vi "AlliGator Phasor Plot Mouse Move Event.vi"(7 "Source Image Display Refnum":T4, 8 "Error In":errorcluster, 9 "Current Phasor Plot Information Indicators":T6, 10 "Image User Event Data":T3, 11 "Alligator Queue Elements in":T1[](array[typedef])) -> (0 "Error Out":errorcluster, 3 "AlliGator Queue Elements out":T1[](array[typedef]))   [LabVIEW 2021, in "AlliGator Phasor Plot.lvlib"]
doc: "Handles mouse move events in the Phasor Plot image."
uses:
  AlliGator Phasor Plot.lvlib
  GUI/AlliGator Phasor Plot Ctrl Refnums.ctl
  Image/Image Control Refnum.ctl
  Image/Image Display User Event Data.ctl
  <vilib>/Utility/miscctls.llb/LVPoint32TypeDef.ctl
  Action Engine/AlliGator Q Element.ctl
  Action Engine/AlliGator Q Event.ctl
  Action Engine/Alligator Elements Order in Action Stack.ctl
  Utilities/Read-Write.ctl
  Phasor Ratio/AlliGator Phasor Reference Data.ctl
  034bdac3-b367-4aff-a885-c1a04e73f031.vi
  034bdac3-b367-4aff-a885-c1a04e73f031.vi/539bd7ec-d9e8-460f-a56d-a449b4a86a5e.vi
  Action Engine/AlliGator Add Action Array to Stack.vi
  Action Engine/AlliGator Action Engine.lvlib
  Phasor Ratio/AlliGator Phasor Ratio.lvlib
  GUI/GUI.lvlib
  Utilities/Utilities.lvlib
  GUI/AlliGator GUI.lvlib
  Image/Image.lvlib
panel:
  # "see the AlliGator License on the block diagram (Ctrl+E or Window:Show Block Diagram)"
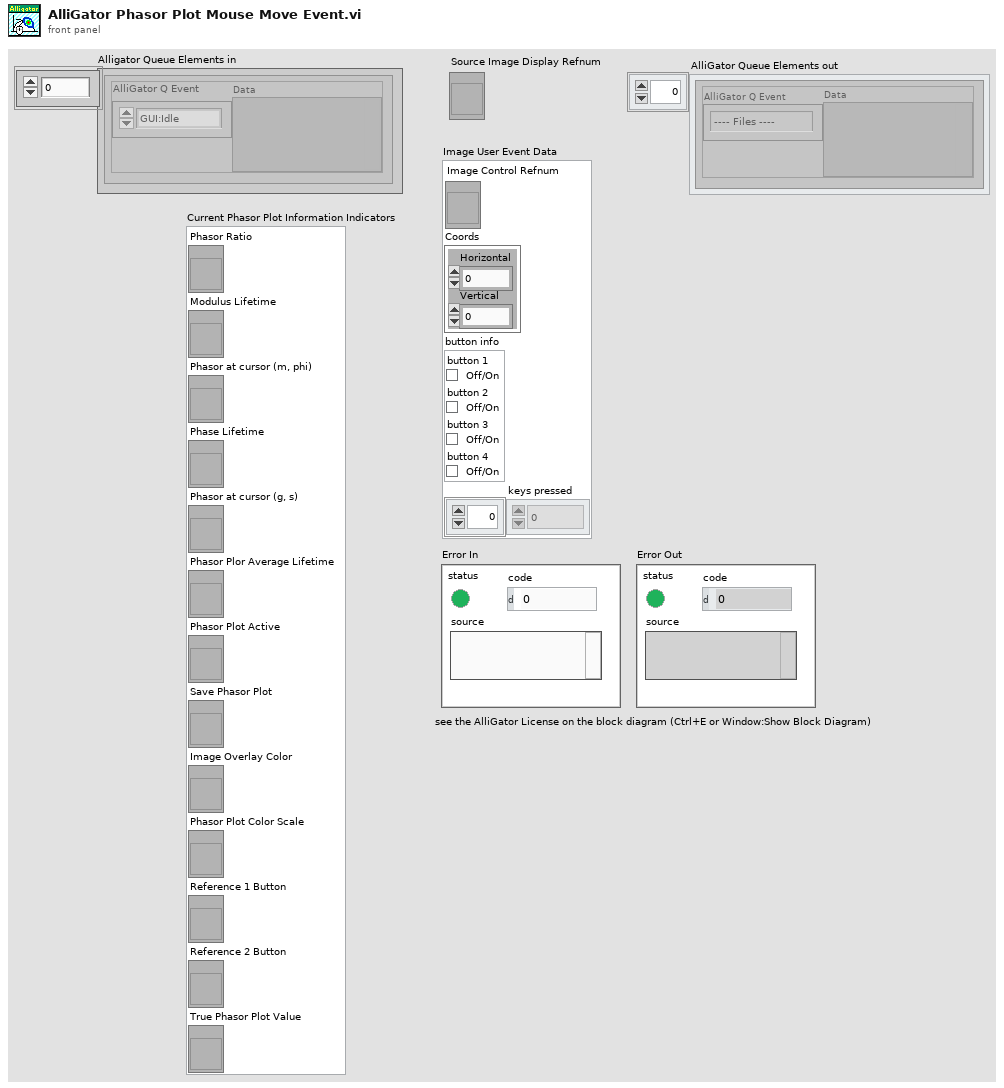
[diagram p1: front panel]
types:
  T1 = typedef "AlliGator Action Engine.lvlib/AlliGator Q Element.ctl" = cluster{"AlliGator Q Event":T2, "Data":variant}
  T2 = typedef "AlliGator Action Engine.lvlib/AlliGator Q Event.ctl" = enum16{"---- Files ----", "Files:Set Batch Export Files To Save", "Files:Set Dataset Loading & Pre-processing Options", "Files:Check #Frames in Dataset", "Files:Increment Frame Index", "Files:Open Mask Image", "Files:Open White Light Image", "Files:Open Single Dataset", "Files:New Folder of Folders Selected", "Files:Load File (all Types)_Scriptable", "Files:Move Flattened Series to Folders Series", "Files:Select Folder", "Files:Load FLI Dataset", "Files:Load Swiss SPAD 1 Dataset", "Files:Load Swiss SPAD 2 Dataset", "Files:Load .sdt FLI Dataset", "Files:Load .ptu FLI Dataset", "Files:Load .bin FLI Dataset", "Files:Load Single Gate Image Folder", "Files:Load I/m/phi Dataset (deprecated)", "Files:Load Single Image", "Files:Subtract Background File", "Files:Export FLI Dataset", "Files:Load HDF5 FLI Dataset", "Files:Set Destination File Path", "Files:Save Mask Image", "Files:Batch Conversion", "Files:New Folder Selected", "Files:Close FLI Dataset", "Files:Close FLI Dataset Series", "Files:Close White Light Image", "Files:Close Mask Image", "---- FLI Dataset ----", "FLI Dataset:Channel Arithmetic", "FLI Dataset:Export Average Lifetime Map as ASCII", "FLI Dataset:Export User-Defined Quantity Map as ASCII", "FLI Dataset:Python Function FLI Dataset Event", "FLI Dataset:ROI Analysis", "FLI Dataset:Tilted Logistic Square Gated IRF Characteristics Map", "FLI Dataset:Logistic Square Gated IRF Characteristics Map", "FLI Dataset:Square Gated IRF Characteristics Map", "FLI Dataset:Multi-ROI Single-Pixel Phasor Analysis", "FLI Dataset:Multi-ROI Single-Pixel NLSF Analysis", "FLI Dataset:All ROIs IRF Extraction", "FLI Dataset:All ROIs Decay Fit Non-Interactive (Fast + Individual IRF)", "FLI Dataset:All ROIs Phasor Analysis", "FLI Dataset:All ROIs Decay Fit", "FLI Dataset:Fluorescence Decay Statistics", "FLI Dataset:Update Decay Statistics Graph", "FLI Dataset:Get Decay from ROI", "FLI Dataset:All ROIs Average Lifetimes", "FLI Dataset:Save/Load Local IRFs", "FLI Dataset:Clear Local IRFs", "FLI Dataset:Phasor Calibration Maps (# Gates Series) Script", "FLI Dataset:Calibrated Phasor Map Series", "---- FLI Dataset Series ----", "FLI Dataset Series:Sum All Datasets in Series", "FLI Dataset Series:Add Dataset to Accumulated Dataset", "FLI Dataset Series:Display Accumulated Dataset", "FLI Dataset Series:Clear Dataset Series Sum", "FLI Dataset Series:Time-Series Analysis (NLSF)", "FLI Dataset Series:Time-Series Analysis (Phasor)", "---- Image ----", "Image:Update Image Profile Plots", "Image:Image Histogram Cursor Move", "Image:Image Histogram", "Image:Image Contrast", "Image:Set Image Histogram Cursor Move Flag", "Image:Clear Image Overlay", "Image:Use ROI as Search Area", "Image:Set ROI Diameter", "Image:Save Image Data as TIFF", "Image:Save Displayed Image with Overlay", "Image:Save Image Overlay Only", "Image:Save Image as Hot Pixel Mask", "Image:Change Source Image Color Palette", "Image:Copy Image to Clipboard", "Image:Source Image ROI Selection", "Image:Delete All ROIs", "Image:Delete All Unselected ROIs", "Image:Delete ROI", "Image:Merge All ROIs", "Image:Store ROI", "Image:Source Image ROI Storage", "Image:Export ROI Description to Notebook", "Image:Save ROI", "Image:Load ROI", "Image:Paste ROI Definition", "Image:Clear ROI", "Image:Identify ROIs in Mask Image", "Image:Create Complementary ROI", "Image:Create Contour ROI", "Image:Create ROI(s) from Pixels with Peak above Min_Scriptable", "Image:Create ROI(s) from Pixels with Intensity above Min_Scriptable", "Image:Compute ROI Statistics", "Image:Delete ROI(s) based on ROI Characteristics", "Image:Create ROI Grid", "Image:ROI to Individual Pixel ROIs", "Image:Python Function Source Image Event", "Image:Show Phasor Calibration Map ROI Centers", "Image:Convert ROI to Mask Image", "Image:Mouse Move", "Image:Mouse Up", "Image:Set Source Image Mouse Move Flag", "Image:Add Scale Bar Overlay", "Image:Delete Existing ROIs Option", "Image:Overlay ROI Median", "Image:Check Current ROI", "Image:Update True Pixel Value", "---- Decay ----", "Decay:Clear IRF/Reference Plot", "Decay:Add Decay to Graph", "Decay:Smoothen Plot", "Decay:Smoothen Plot Tail", "Decay:Average Selected Plots", "Decay:Extract IRF", "Decay:Optimal IRF Extraction", "Decay:Threshold IRF", "Decay:Fit to Model IRF", "Decay:Fit IRF to Square Gate", "Decay:Fit IRF to Logistic Square Gate", "Decay:Fit IRF to Tilted Logistic Square Gate", "Decay:Create Bounding Cursors Set", "Decay:Export Bounding Cursors Definition to Notebook", "Decay:Denoise Plot", "Decay:Compute Cumulative Function", "Decay:Use as Reference Decay", "Decay:Show Reference Decay/IRF", "Decay:Extrapolate Decay", "Decay:Create Head & Tail Bounding Cursors", "Decay:Store Cursor-defined Head & Tail Fractions", "Decay:Rebin Plot", "Decay:1-Normalize Decay", "Decay:[0-1]-Normalize Plot", "Decay:Straighten Decay", "Decay:Shift Decay", "Decay:Fold Decay", "Decay:Fit Decay", "Decay:Global Fit of Selected Decays", "Decay:Post Global Fit Script", "Decay:Add Global Fit Parameters to Graph", "Decay:Add Decay Parameter(s) to Plot (Graph)", "Decay:Export Decay to Phasor Graph", "Decay:Compute Average Lifetime", "Decay:Plot Convolution", "Decay:Graph Tip Strip Update", "---- Decay Statistics ----", "Decay Statistics:Tip Strip Update", "---- Intensity Time Trace ----", "Intensity Time Trace:Use File Timestamp", "Intensity Time Trace:Load Intensity Corrections File", "Intensity Time Trace:Clear Intensity Corrections File", "Intensity Time Trace:Tip Strip Update", "---- Phasor Plot ----", "Phasor Plot:Build Phasor Plot", "Phasor Plot:Change Phasor Plot Color Palette", "Phasor Plot:Adjust Phasor Plot Display Range", "Phasor Plot:Highlight Image ROI in Phasor Plot", "Phasor Plot:Save Phasor Plot Image with Overlay", "Phasor Plot:Export Complex Phasor Map", "Phasor Plot:Export Phasor Ratio Map", "Phasor Plot:Export Average Lifetime Map", "Phasor Plot:Compute Phase Lifetime Histogram", "Phasor Plot:Compute Phasor Ratio Histogram", "Phasor Plot:Compute Phase Lifetime vs Intensity Scatter Plot", "Phasor Plot:Weber 2-Component Decomposition", "Phasor Plot:Update Phasor Color Map Vertices", "Phasor Plot:Clear Phasor Overlay", "Phasor Plot:Use Segment Extremities as References", "Phasor Plot:Use UC/Segment Intersections as References", "Phasor Plot:Use UC/Principal Axis Intersections as References", "Phasor Plot:Use UC/Linear Fit Intersections as References", "Phasor Plot:Update Phasor Plot Reference", "Phasor Plot:Show Local Phasor Info in Phasor Plot", "Phasor Plot:Update Phasor Plot State", "Phasor Plot:Phasor Plot ROI Storage", "Phasor Plot:Phasor Plot ROI Selection", "Phasor Plot:Python Function Phasor Plot Event", "Phasor Plot:Overlay Phasor ROI, Ratio or Map in Source Image", "Phasor Plot:Compute Decay of Selected Phasors", "Phasor Plot:Phasor at Image Pixel", "Phasor Plot:Mouse Move", "Phasor Plot:Mouse Up", "Phasor Plot:Display Range Mouse Move", "Phasor Plot:Set Mouse Move Flag", "Phasor Plot:Update True Phasor Plot Value", "---- Phasor Graph ----", "Phasor Graph:Get Phasor Value", "Phasor Graph:Create New Phasor Plot Dialog", "Phasor Graph:Update Last Phasor Value", "Phasor Graph:Update Phasor (m, phi)", "Phasor Graph:Remove Single Phasor from Plot", "Phasor Graph:Add Single Phasor to Plot", "Phasor Graph:Remove Phasor Plot", "Phasor Graph:Remove Selected Phasor Plots", "Phasor Graph:Clear Phasor Data", "Phasor Graph:Clear Phasor Graph", "Phasor Graph:Cursor Move", "Phasor Graph:Draw Cursor Connecting Line", "Phasor Graph:Clear Cursor Connecting Line", "Phasor Graph:Find UC Intersection", "Phasor Graph:Use UC/Cursor-Defined Line Intersections", "Phasor Graph:Use Selected Plots Fitted Line/UC Intersections", "Phasor Graph:Use Selected Plots Principal Axis/UC Intersections", "Phasor Graph:Show Single Phasor", "Phasor Graph:Save Single Phasor Plot", "Phasor Graph:Save All Phasor Plots", "Phasor Graph:Load Phasor Plot(s)", "Phasor Graph:Phasor Multiplication", "Phasor Graph:Compute Average Phasor", "Phasor Graph:Compute Multiple Average Phasors (Selected Plots)", "Phasor Graph:Export Single Phasor Plot Phase Lifetimes", "Phasor Graph:Parameter 2 vs Parameter 1 Scatter Plot", "Phasor Graph:Use Cursor n Location", "Phasor Graph:Set Reference n to Current Phase Lifetime Value", "Phasor Graph:Set Reference n to Lifetime Value", "Phasor Graph:Set Cursor n Location", "Phasor Graph:Save Phasor Graph Image", "Phasor Graph:Update SEPL Plot", "Phasor Graph:Export Single Phasor Plot Data", "Phasor Graph:Export Selected Phasor Plots Data", "Phasor Graph:Python Function Phasor Graph Event", "Phasor Graph:Tip Strip Update", "---- Calibration ----", "Calibration:Set Calibration Type", "Calibration:Load/Save Phasor Calibration", "Calibration:Load/Save Phasor Calibration Series", "Calibration:Load/Save Phasor Calibration Map", "Calibration:Use as Calibration", "Calibration:Compute Optimal Calibration from Phasor References", "Calibration:Clear Phasor Calibration", "Calibration:Single Phasor Calibration Information", "Calibration:Use as Calibration Series", "Calibration:Use as Calibration Map", "Calibration:Clear Calibration Series", "Calibration:Phasor Calibration Series Information", "Calibration:Clear Calibration Map", "Calibration:Phasor Calibration Map Information", "Calibration:Apply Phasor Calibration", "Calibration:Update Single Plot Calibration", "Calibration:Update Multiple Plots Calibration", "Calibration:Clear Single Plot Calibration", "Calibration:Clear All Plots Calibrations", "Calibration:Clear Plot(s) Calibration(s)?", "---- Phasor Ratio ----", "Phasor Ratio:Clear Reference n", "Phasor Ratio:Toggle Selected Plot(s)  Lock to Reference 1", "Phasor Ratio:Use as Reference n", "Phasor Ratio:Send Reference n to Notebook", "Phasor Ratio:Toggle Selected Plot(s)  Lock to Reference 2", "Phasor Ratio:Compute Phasor Ratio at Mouse Location", "Phasor Ratio:Compute Phasor Plot's Average Phasor Ratio", "Phasor Ratio:Compute Time-Series Phasor Ratios", "Phasor Ratio:Fit Line to Phasor Ratio Plot", "Phasor Ratio:Save References", "Phasor Ratio:Load References", "Phasor Ratio:Update Phasor Reference 1", "Phasor Ratio:Update Phasor Reference 2", "Phasor Ratio:Move Cursor n to Reference n", "Phasor Ratio:Use as Phasor Reference 1 Lifetime", "Phasor Ratio:Use as Phasor Reference 2 Lifetime", "Phasor Ratio:Export Phasor Ratio Map as ASCII", "Phasor Ratio:Tip Strip Update", "---- Lifetime & Other Parameters Graph ----", "Lifetime:Compute Sliced Mean, SDV and CV Plots", "Lifetime:Plot Decay Shifts", "Lifetime:Plot Histogram", "---- Decay Fit Parameter Map ----", "Decay Fit Parameter Map:Export ROI NLSF Data as ASCII", "Decay Fit Parameter Map:Set Decay Fit Parameter Map Selection", "Decay Fit Parameter Map:Build Decay Fit Parameter Map", "Decay Fit Parameter Map:Change Decay Fit Parameter Map Color Palette", "Decay Fit Parameter Map:Export Decay Fit Parameter Map Data as ASCII", "Decay Fit Parameter Map:Export All Decay Fit Parameter Maps Data as ASCII", "Decay Fit Parameter Map:Selected Parameter Scatterplot", "Decay Fit Parameter Map:Parameter 2 vs Parameter 1 Scatterplot", "Decay Fit Parameter Map:Save Decay Fit Parameter Map Image", "Decay Fit Parameter Map:Save-Load IRFs & Fit Data", "Decay Fit Parameter Map:Update Local Decay Plots", "Decay Fit Parameter Map:Python Function Decay Fit Parameters Map Event", "Decay Fit Parameter Map:Overlay Decay Fit Parameter Map in Source Image", "Decay Fit Parameter Map:Selected Parameter vs Intensity Scatterplot", "Decay Fit Parameter Map:Mouse Up", "Decay Fit Parameter Map:Mouse Move", "Decay Fit Parameter Map:Display Range Mouse Move", "Decay Fit Parameter Map:Change Map Resolution", "Decay Fit Parameter Map:Variance Significance Maps", "Decay Fit Parameter Map:Fit Result Constraints Window", "---- Parameter Map ----", "Parameter Map:Export ROI Parameters Data as ASCII", "Parameter Map:Add Parameter Map Set", "Parameter Map:Delete Parameter Map Set", "Parameter Map:Update Parameter List", "Parameter Map:Build Parameter Map", "Parameter Map:Change Parameter Map Color Palette", "Parameter Map:Export Parameter Map Data as ASCII", "Parameter Map:Export All Parameter Maps Data as ASCII", "Parameter Map:Selected Parameter Scatterplot", "Parameter Map:Parameter 2 vs Parameter 1 Scatterplot", "Parameter Map:Selected Parameter vs Intensity Scatterplot", "Parameter Map:Save Parameter Map Image", "Parameter Map:Save-Load IRFs & Parameter Maps (TODO)", "Parameter Map:Set Parameter Map Selection", "Parameter Map:Python Function Parameter Map Event", "Parameter Map:Overlay Parameter Map in Source Image", "Parameter Map:Update Local Decay Plots", "Parameter Map:Mouse Up", "Parameter Map:Mouse Move", "Parameter Map:Display Range Mouse Move", "---- Generic Graph ----", "Generic Graph:Generic XY Graph Event", "Generic Graph:Python Function XY Graph Event", "Generic Graph:New Plot", "Generic Graph:Save Plot", "Generic Graph:XY Plot Histogram", "Generic Graph:Set XY Graph Plot Name", "Generic Graph:Set Last Cursor Style", "Generic Graph:Tip Strip Update", "---- GUI ----", "GUI:Start Script", "GUI:Type of Displayed Image Changed", "GUI:Gate Image Slide Changed", "GUI:Show Busy Icon", "GUI:Show Busy Icon & Abort Button", "GUI:Hide Busy Icon", "GUI:Hide Busy Icon & Abort Button", "GUI:Abort", "GUI:End Script", "GUI:Start Timing", "GUI:End Timing", "GUI:Set State Indicator", "GUI:Send Parameters JSON Strings to Clipboard", "GUI:Set Gate Step", "GUI:Idle", "GUI:Initialization", "GUI:Quit", "GUI:Increment Dataset Index", "GUI:Set Dataset Index to -1", "GUI:Time Series Slider Moved", "GUI:Time Series Slider Changed", "GUI:Toggle Playback or Loop", "GUI:Playback Script", "GUI:Set Phasor Frequency", "GUI:Open Window", "GUI:Start Test Script", "GUI:End Test Script", "GUI:Set Verbose Mode", "GUI:Set Verbose Settings Mode", "DEBUG"}
  T3 = typedef "Image.lvlib/Image Display User Event Data.ctl" = cluster{"Image Control Refnum":T4, "Coords":T5, "button info":cluster{"button 1":bool, "button 2":bool, "button 3":bool, "button 4":bool}, "keys pressed":enum16{"0", "1", "2", "3", "4", "5", "6", "7", "8", "9", "A", "B", "C", "D", "E", "F", "G", "H", "I", "J", "K", "L", "M", "N", "O", "P", "Q", "R", "S", "T", "U", "V", "W", "X", "Y", "Z", "F1", "F2", "F3", "F4", "F5", "F6", "F7", "F8", "F9", "F10", "F11", "F12", "F13", "F14", "F15", "ADD", "BACK", "BACKSLASH", "CAPITAL", "COMMA", "DECIMAL", "DELETE", "DIVIDE", "DOWN", "END", "EQUALS", "ESCAPE", "GRAVE (`)", "HOME", "INSERT", "LBRACKET", "LCONTROL", "LEFT", "L ALT", "LSHIFT", "LWIN", "MINUS", "MULTIPLY", "NEXT", "NUMLOCK", "NUMPAD_0", "NUMPAD_1", "NUMPAD_2", "NUMPAD_3", "NUMPAD_4", "NUMPAD_5", "NUMPAD_6", "NUMPAD_7", "NUMPAD_8", "NUMPAD_9", "PAUSE", "PERIOD", "PRIOR (PG UP)", "RBRACKET", "RCONTROL", "RETURN", "RIGHT", "R ALT", "RSHIFT", "RWIN", "SCROLL", "SEMICOLON", "SLASH", "SPACE", "SUBTRACT", "TAB", "UP", "ENTER (num pad)", "' (quote)"}[]}
  T4 = typedef "Image.lvlib/Image Control Refnum.ctl" = refnum<vi>
  T5 = typedef "LVPoint32TypeDef.ctl" = cluster{"Horizontal":i32, "Vertical":i32}
  T6 = typedef "AlliGator GUI.lvlib/AlliGator Phasor Plot Ctrl Refnums.ctl" = cluster{"Phasor Ratio":refnum<vi>, "Modulus Lifetime":refnum<vi>, "Phasor at cursor (m, phi)":refnum<vi>, "Phase Lifetime":refnum<vi>, "Phasor at cursor (g, s)":refnum<vi>, "Phasor Plor Average Lifetime":refnum<vi>, "Phasor Plot Active":refnum<vi>, "Save Phasor Plot":refnum<vi>, "Image Overlay Color":refnum<vi>, "Phasor Plot Color Scale":refnum<vi>, "Reference 1 Button":refnum<vi>, "Reference 2 Button":refnum<vi>, "True Phasor Plot Value":refnum<vi>}
  T7 = typedef "AlliGator Action Engine.lvlib/Alligator Elements Order in Action Stack.ctl" = enum16{"Enqueue 2 AFTER 1", "Enqueue 2 BEFORE 1"}
  T8 = enum16{"0", "1", "2", "3", "4", "5", "6", "7", "8", "9", "A", "B", "C", "D", "E", "F", "G", "H", "I", "J", "K", "L", "M", "N", "O", "P", "Q", "R", "S", "T", "U", "V", "W", "X", "Y", "Z", "F1", "F2", "F3", "F4", "F5", "F6", "F7", "F8", "F9", "F10", "F11", "F12", "F13", "F14", "F15", "ADD", "BACK", "BACKSLASH", "CAPITAL", "COMMA", "DECIMAL", "DELETE", "DIVIDE", "DOWN", "END", "EQUALS", "ESCAPE", "GRAVE (`)", "HOME", "INSERT", "LBRACKET", "LCONTROL", "LEFT", "L ALT", "LSHIFT", "LWIN", "MINUS", "MULTIPLY", "NEXT", "NUMLOCK", "NUMPAD_0", "NUMPAD_1", "NUMPAD_2", "NUMPAD_3", "NUMPAD_4", "NUMPAD_5", "NUMPAD_6", "NUMPAD_7", "NUMPAD_8", "NUMPAD_9", "PAUSE", "PERIOD", "PRIOR (PG UP)", "RBRACKET", "RCONTROL", "RETURN", "RIGHT", "R ALT", "RSHIFT", "RWIN", "SCROLL", "SEMICOLON", "SLASH", "SPACE", "SUBTRACT", "TAB", "UP", "ENTER (num pad)", "' (quote)"}[]
  T9 = enum16{"0", "1", "2", "3", "4", "5", "6", "7", "8", "9", "A", "B", "C", "D", "E", "F", "G", "H", "I", "J", "K", "L", "M", "N", "O", "P", "Q", "R", "S", "T", "U", "V", "W", "X", "Y", "Z", "F1", "F2", "F3", "F4", "F5", "F6", "F7", "F8", "F9", "F10", "F11", "F12", "F13", "F14", "F15", "ADD", "BACK", "BACKSLASH", "CAPITAL", "COMMA", "DECIMAL", "DELETE", "DIVIDE", "DOWN", "END", "EQUALS", "ESCAPE", "GRAVE (`)", "HOME", "INSERT", "LBRACKET", "LCONTROL", "LEFT", "L ALT", "LSHIFT", "LWIN", "MINUS", "MULTIPLY", "NEXT", "NUMLOCK", "NUMPAD_0", "NUMPAD_1", "NUMPAD_2", "NUMPAD_3", "NUMPAD_4", "NUMPAD_5", "NUMPAD_6", "NUMPAD_7", "NUMPAD_8", "NUMPAD_9", "PAUSE", "PERIOD", "PRIOR (PG UP)", "RBRACKET", "RCONTROL", "RETURN", "RIGHT", "R ALT", "RSHIFT", "RWIN", "SCROLL", "SEMICOLON", "SLASH", "SPACE", "SUBTRACT", "TAB", "UP", "ENTER (num pad)", "' (quote)"}
  T10 = typedef "Utilities.lvlib/Read-Write.ctl" = enum16{"Read", "Write"}
  T11 = typedef "AlliGator Phasor Ratio.lvlib/AlliGator Phasor Reference Data.ctl" = cluster{"Data Type":string, "Data":variant}
  T12 = typedef "IMAQ Image.ctl" = refnum<image>
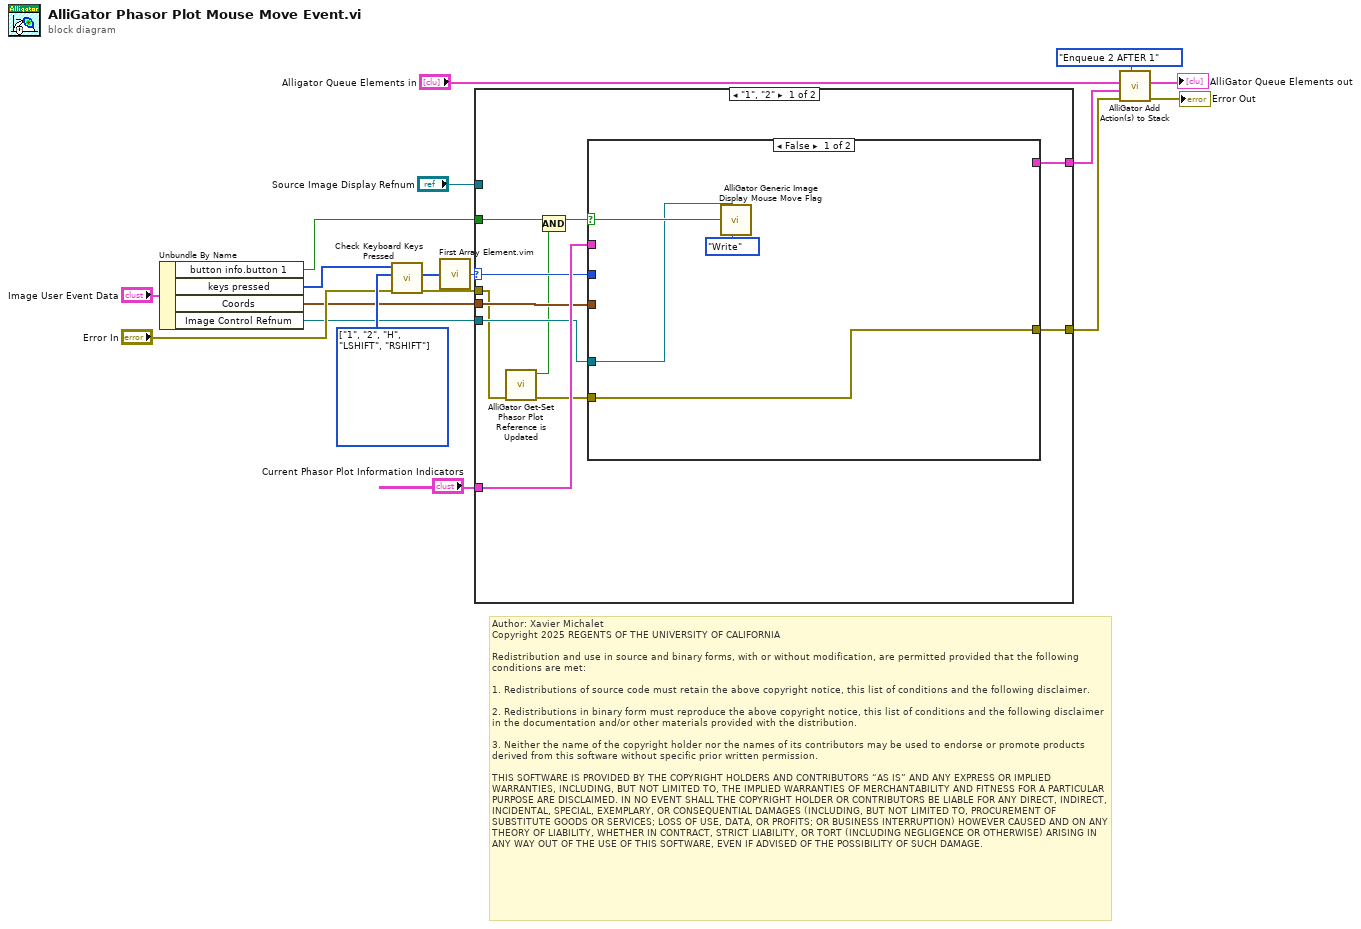
[diagram p0: block diagram]
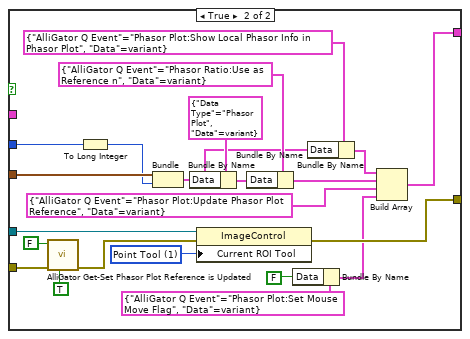
[diagram p2: hidden frame]
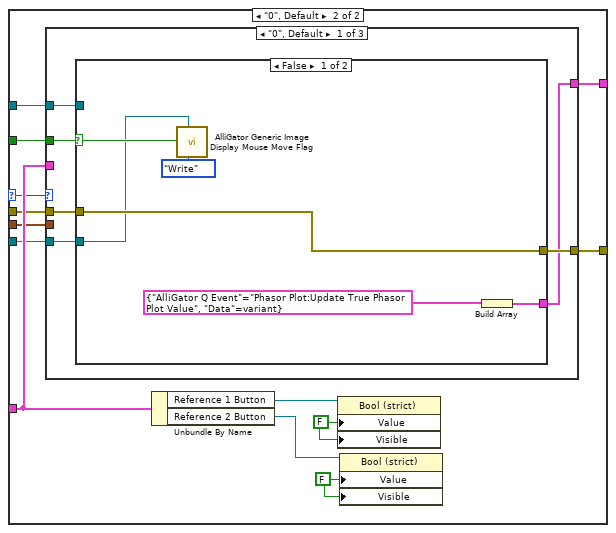
[diagram p3: hidden frame]
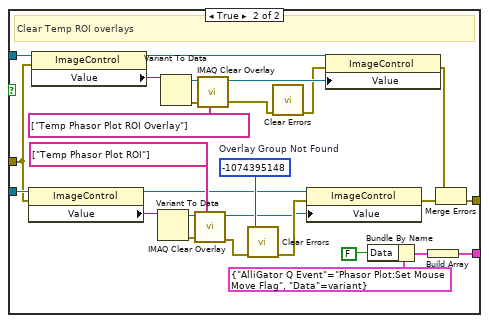
[diagram p4: hidden frame]
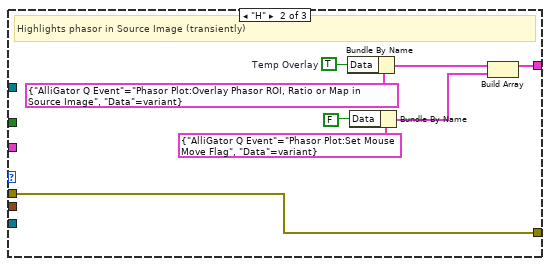
[diagram p5: hidden frame]
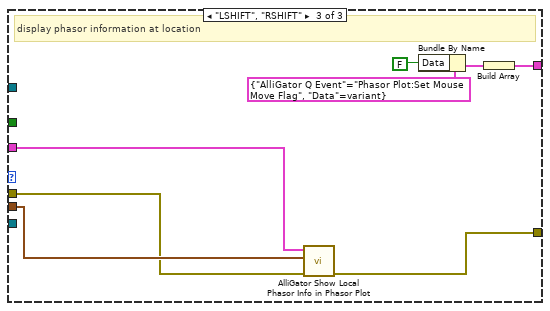
[diagram p6: hidden frame]
diagram:
  w17 = T8 [enum."1", enum."2", enum."H", enum."LSHIFT", enum."RSHIFT"] items=["0", "1", "2", "3", "4", "5", "6", "7", "8", "9", "A", "B", "C", "D", "E", "F", "G", "H", "I", "J", "K", "L", "M", "N", "O", "P", "Q", "R", "S", "T", "U", "V", "W", "X", "Y", "Z", "F1", "F2", "F3", "F4", "F5", "F6", "F7", "F8", "F9", "F10", "F11", "F12", "F13", "F14", "F15", "ADD", "BACK", "BACKSLASH", "CAPITAL", "COMMA", "DECIMAL", "DELETE", "DIVIDE", "DOWN", "END", "EQUALS", "ESCAPE", "GRAVE (`)", "HOME", "INSERT", "LBRACKET", "LCONTROL", "LEFT", "L ALT", "LSHIFT", "LWIN", "MINUS", "MULTIPLY", "NEXT", "NUMLOCK", "NUMPAD_0", "NUMPAD_1", "NUMPAD_2", "NUMPAD_3", "NUMPAD_4", "NUMPAD_5", "NUMPAD_6", "NUMPAD_7", "NUMPAD_8", "NUMPAD_9", "PAUSE", "PERIOD", "PRIOR (PG UP)", "RBRACKET", "RCONTROL", "RETURN", "RIGHT", "R ALT", "RSHIFT", "RWIN", "SCROLL", "SEMICOLON", "SLASH", "SPACE", "SUBTRACT", "TAB", "UP", "ENTER (num pad)", "' (quote)"] ("key targets (all)")
  # "Author: Xavier Michalet\nCopyright 2025 REGENTS OF THE UNIVERSITY OF CALIFORNIA\n\nRedistribution and use in source and binary forms, with or without modification, are permitted provided that the following conditions are met:\n\n1. Redistributions of source code must retain the above copyright notice, this list of conditions and the following disclaimer.\n\n2. Redistributions in binary form must reproduce the above copyright notice, this list of conditions and the following disclaimer in the documentation and/or other materials provided with the distribution.\n\n3. Neither the name of the copyright holder nor the names of its contributors may be used to endorse or promote products derived from this software without specific prior written permission.\n\nTHIS SOFTWARE IS PROVIDED BY THE COPYRIGHT HOLDERS AND CONTRIBUTORS “AS IS” AND ANY EXPRESS OR IMPLIED WARRANTIES, INCLUDING, BUT NOT LIMITED TO, THE IMPLIED WARRANTIES OF MERCHANTABILITY AND FITNESS FOR A PARTICULAR PURPOSE ARE DISCLAIMED. IN NO EVENT SHALL THE COPYRIGHT HOLDER OR CONTRIBUTORS BE LIABLE FOR ANY DIRECT, INDIRECT, INCIDENTAL, SPECIAL, EXEMPLARY, OR CONSEQUENTIAL DAMAGES (INCLUDING, BUT NOT LIMITED TO, PROCUREMENT OF SUBSTITUTE GOODS OR SERVICES; LOSS OF USE, DATA, OR PROFITS; OR BUSINESS INTERRUPTION) HOWEVER CAUSED AND ON ANY THEORY OF LIABILITY, WHETHER IN CONTRACT, STRICT LIABILITY, OR TORT (INCLUDING NEGLIGENCE OR OTHERWISE) ARISING IN ANY WAY OUT OF THE USE OF THIS SOFTWARE, EVEN IF ADVISED OF THE POSSIBILITY OF SUCH DAMAGE."
  n1 = Unbundle By Name("Image User Event Data") -> ("button info.button 1"=w10:bool, "keys pressed"=w9:T8, "Coords"=w8:T5, "Image Control Refnum"=w7:T4)
  n2 = call "Check Keyboard Keys Pressed.vi"("error in (no error)"="Error In", "key targets (all)"=w17, "keys pressed"=w9) -> ("error out"=w13:errorcluster, "keys found"=w15:T8)  [unwired: 6 in, 1 out]
  n3 = call "First Array Element.vim"("Array"=w15) -> ("First Element"=w16:T9)  [unwired: 8 in]
  n4 = case shown="\"1\", \"2\"" w16 {
    selector: w16 -> [w24 w62]
    tunnel: [w29 w68] -> w4
    tunnel: "Current Phasor Plot Information Indicators" -> [w28 w67]
    tunnel: w13 -> [w22 w66]
    tunnel: w7 -> [w27 w65]
    tunnel: w8 -> [w26 w64]
    tunnel: w10 -> [w25 w63]
    tunnel: "Source Image Display Refnum" -> [_ w61]
    tunnel: [w23 w60] -> w6
    frame "1", "2" {
      n5 = call "AlliGator Get-Set Phasor Plot Reference is Updated.vi"("error in (no error)"=w22) -> ("error out"=w21:errorcluster, "Phasor Plot Reference Updated ?"=w19:bool)  [unwired: 9 in]
      n6 = Compound Arithmetic op=AND(w25, w19) -> (w20:bool)
      n7 = case shown="False" w20 {
        selector: w20 -> [w31 _]
        tunnel: w24 -> [_ w42]
        tunnel: w26 -> [_ w45]
        tunnel: [_ w50] -> w23
        tunnel: w27 -> [w30 w48]
        tunnel: w21 -> [w33 w40]
        tunnel: [w33 w44] -> w29
        tunnel: w28 -> [_ _]
        frame False {
          n8 = call "AlliGator Generic Image Display Mouse Move Flag.vi"("Image Control Refnum"=w30, "Flag (in)"=w31, "Read/Write"=Read-Write."Write") -> ()  [unwired: 6 in, 1 out]
        }
        frame True {
          w49 = u32 1 items=["Zoom Tool"=8, "Selection Tool"=0, "Pan Tool"=9, "Point Tool"=1, "Line Tool"=2, "Rectangle Tool"=3, "Rotated Rectangle Tool"=12, "Polyline Tool"=10, "Polygon Tool"=5, "Freehand Tool"=11, "Closed Freehand Tool"=6, "Ellipse Tool"=4, "Annulus Tool"=7] ("Current ROI Tool")
          n9 = call "AlliGator Get-Set Phasor Plot Reference is Updated.vi"("Set/Get (F)"=TRUE, "error in (no error)"=w40, "Phasor Plot Reference Updated"=FALSE) -> ("error out"=w37:errorcluster)  [unwired: 7 in, 1 out]
          n10 = To Long Integer(number=w42) -> (32bit integer=w41:i32)
          n11 = Bundle("Coords"=w45, w41) -> (w43:cluster{"Coords":T5, i32})  [unwired: 1 in]
          n12 = Bundle By Name(cluster=T11 {"Data Type"="Phasor Plot", "Data"=variant} ("Phasor Reference Data"), "Data"=w43) -> (w54:T11)
          n13 = property class="ImageControl"(reference=w48, error in=w37, "Current ROI Tool"=w49) -> (error out=w44:errorcluster)  [unwired: 1 out]
          n14 = Bundle By Name(cluster=T1 {"AlliGator Q Event"=enum."Phasor Ratio:Use as Reference n", "Data"=variant} ("Time-Gated Phasor Q Element"), "Data"=w54) -> (w53:T1)
          n15 = Bundle By Name(cluster=T1 {"AlliGator Q Event"=enum."Phasor Plot:Set Mouse Move Flag", "Data"=variant} ("element"), "Data"=FALSE) -> (w34:T1)
          n16 = Bundle By Name(cluster=T1 {"AlliGator Q Event"=enum."Phasor Plot:Show Local Phasor Info in Phasor Plot", "Data"=variant} ("element"), "Data"=w43) -> (w46:T1)
          n17 = Build Array(w46, w53, T1 {"AlliGator Q Event"=enum."Phasor Plot:Update Phasor Plot Reference", "Data"=variant} ("Time-Gated Phasor Q Element"), w34) -> (w50:T1[])
        }
      }
    }
    frame "0", Default {
      w57 = FALSE ("Value")
      w56 = FALSE ("Value")
      n18 = case shown="\"0\", Default" w62 {
        tunnel: w64 -> [_ _ w123]
        tunnel: [w69 w111 w116] -> w60
        tunnel: w65 -> [w72 _ _]
        tunnel: w66 -> [w73 w115 w121]
        tunnel: [w71 w115 w120] -> w68
        tunnel: w67 -> [_ _ w122]
        tunnel: w63 -> [w74 _ _]
        tunnel: w61 -> [w70 _ _]
        frame "0", Default {
          n19 = case shown="False" w74 {
            selector: w74 -> [w78 _]
            tunnel: w73 -> [w80 w90]
            tunnel: w72 -> [w75 w107]
            tunnel: [w80 w87] -> w71
            tunnel: w70 -> [_ w91]
            tunnel: [w76 w81] -> w69
            frame False {
              n20 = call "AlliGator Generic Image Display Mouse Move Flag.vi"("Image Control Refnum"=w75, "Flag (in)"=w78, "Read/Write"=Read-Write."Write") -> ()  [unwired: 6 in, 1 out]
              n21 = Build Array(T1 {"AlliGator Q Event"=enum."Phasor Plot:Update True Phasor Plot Value", "Data"=variant}) -> (w76:T1[])
            }
            frame True {
              w101 = -1074395148  # Overlay Group Not Found
              # "Clear Temp ROI overlays"
              n22 = property class="ImageControl"(reference=w107, error in=w90) -> (reference out=w100:T4, "Value"=w106:variant)  [unwired: 1 out]
              n23 = property class="ImageControl"(reference=w91, error in=w90) -> (reference out=w95:T4, "Value"=w92:variant)  [unwired: 1 out]
              n24 = Variant To Data(Variant=w106) -> (data=w105:T12, error out=w104:errorcluster)  [unwired: 2 in]
              n25 = Variant To Data(Variant=w92) -> (data=w93:T12, error out=w94:errorcluster)  [unwired: 2 in]
              n26 = call "IMAQ Clear Overlay"("Groups"=string[] ["Temp Phasor Plot ROI"], "error in (no error)"=w104, "Image"=w105) -> ("error out"=w102:errorcluster, "Image Out"=w98:T12)  [unwired: 7 in]
              n27 = call "IMAQ Clear Overlay"("Groups"=string[] ["Temp Phasor Plot ROI Overlay"], "error in (no error)"=w94, "Image"=w93) -> ("error out"=w89:errorcluster, "Image Out"=w96:T12)  [unwired: 7 in]
              n28 = call <vilib>:"Clear Errors.vi"("error in (no error)"=w102, "specific error code to clear (0: all)"=w101) -> ("error out"=w99:errorcluster)  [unwired: 4 in, 1 out]
              n29 = call <vilib>:"Clear Errors.vi"("error in (no error)"=w89) -> ("error out"=w88:errorcluster)  [unwired: 5 in, 1 out]
              n30 = property class="ImageControl"(reference=w100, error in=w99, "Value"=w98) -> (error out=w97:errorcluster)  [unwired: 1 out]
              n31 = property class="ImageControl"(reference=w95, error in=w88, "Value"=w96) -> (error out=w86:errorcluster)  [unwired: 1 out]
              n32 = Bundle By Name(cluster=T1 {"AlliGator Q Event"=enum."Phasor Plot:Set Mouse Move Flag", "Data"=variant} ("element"), "Data"=FALSE) -> (w82:T1)
              n33 = Build Array(w82) -> (w81:T1[])
              n34 = Merge Errors(w86, w97) -> (w87:errorcluster)
            }
          }
        }
        frame "H" {
          w112 = TRUE  # Temp Overlay
          # "Highlights phasor in Source Image (transiently)"
          n35 = Bundle By Name(cluster=T1 {"AlliGator Q Event"=enum."Phasor Plot:Overlay Phasor ROI, Ratio or Map in Source Image", "Data"=variant} ("Time-Gated Phasor Q Element"), "Data"=w112) -> (w113:T1)
          n36 = Bundle By Name(cluster=T1 {"AlliGator Q Event"=enum."Phasor Plot:Set Mouse Move Flag", "Data"=variant} ("element"), "Data"=FALSE) -> (w108:T1)
          n37 = Build Array(w113, w108) -> (w111:T1[])
        }
        frame "LSHIFT", "RSHIFT" {
          # "display phasor information at location"
          n38 = call "AlliGator Show Local Phasor Info in Phasor Plot.vi"("error in (no error)"=w121, "Last Mouse Position"=w123, "Current Phasor Plot Information Indicators"=w122) -> ("error out"=w120:errorcluster)  [unwired: 8 in]
          n39 = Bundle By Name(cluster=T1 {"AlliGator Q Event"=enum."Phasor Plot:Set Mouse Move Flag", "Data"=variant} ("element"), "Data"=FALSE) -> (w117:T1)
          n40 = Build Array(w117) -> (w116:T1[])
        }
      }
      n41 = Unbundle By Name(w67) -> ("Reference 1 Button"=w58:refnum<vi>, "Reference 2 Button"=w59:refnum<vi>)
      n42 = property class="Bool (strict)"(reference=w58, "Value"=w56, "Visible"=w56) -> ()  [unwired: 1 in, 2 out]
      n43 = property class="Bool (strict)"(reference=w59, "Value"=w57, "Visible"=w57) -> ()  [unwired: 1 in, 2 out]
    }
  }
  n44 = call-poly "AlliGator Add Action(s) to Stack.vi"("Elements Order in Action Stack (Default: 2 BEFORE 1)"=Alligator_Elements_Order_in_Action_Stack."Enqueue 2 AFTER 1", "Error In"=w4, "Alligator Queue Element 2"=w6, "Alligator Queue Element 1"="Alligator Queue Elements in") -> ("Error Out"=→"Error Out":errorcluster, "Alligator Queue Element 1 (+ 2)"=→"AlliGator Queue Elements out":T1[])  [unwired: 6 in]
